vi "BRig_RT__Case_Exp__State_initTrial2__v3.vi"(0 "input_dataCurrent":u16[](array[numeric]), 1 "input_dataTrial":u16[][](array[numeric]), 3 "input_dataExp":u16[](array[numeric]), 6 "input_dataBlock":u16[][](array[numeric]), 8 "input_dataLC":u16[](array[numeric])) -> (7 "output_L_Wrong_Laser_l2":bool, 9 "output_L_Wrong_Event_l2":bool, 10 "output_L_Power_l1":dbl, 11 "output_L_Reward_Laser_l2":bool, 12 "output_L_Power_l2":dbl, 13 "output_L_Reward_Event_l2":bool, 14 "output_dataCurrent":u16[](array[numeric]), 15 "output_dataTrial":u16[][](array[numeric]), 16 "output_L_Reward_Event_l1":bool, 17 "output_L_Reward_Laser_l1":bool, 18 "output_L_Wrong_Event_l1":bool, 19 "output_L_Wrong_Laser_l1":bool)   [LabVIEW 2014]
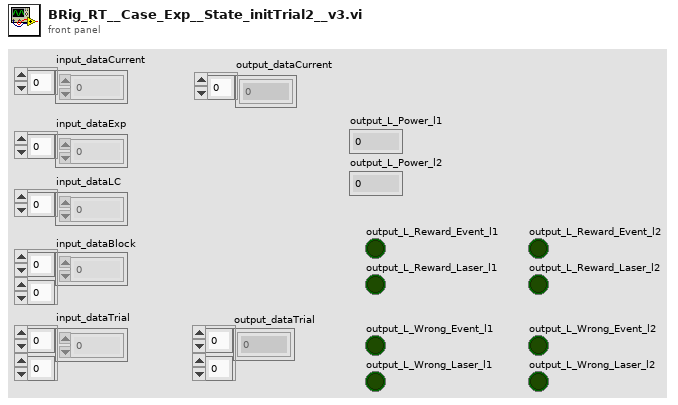
[diagram p1: front panel]
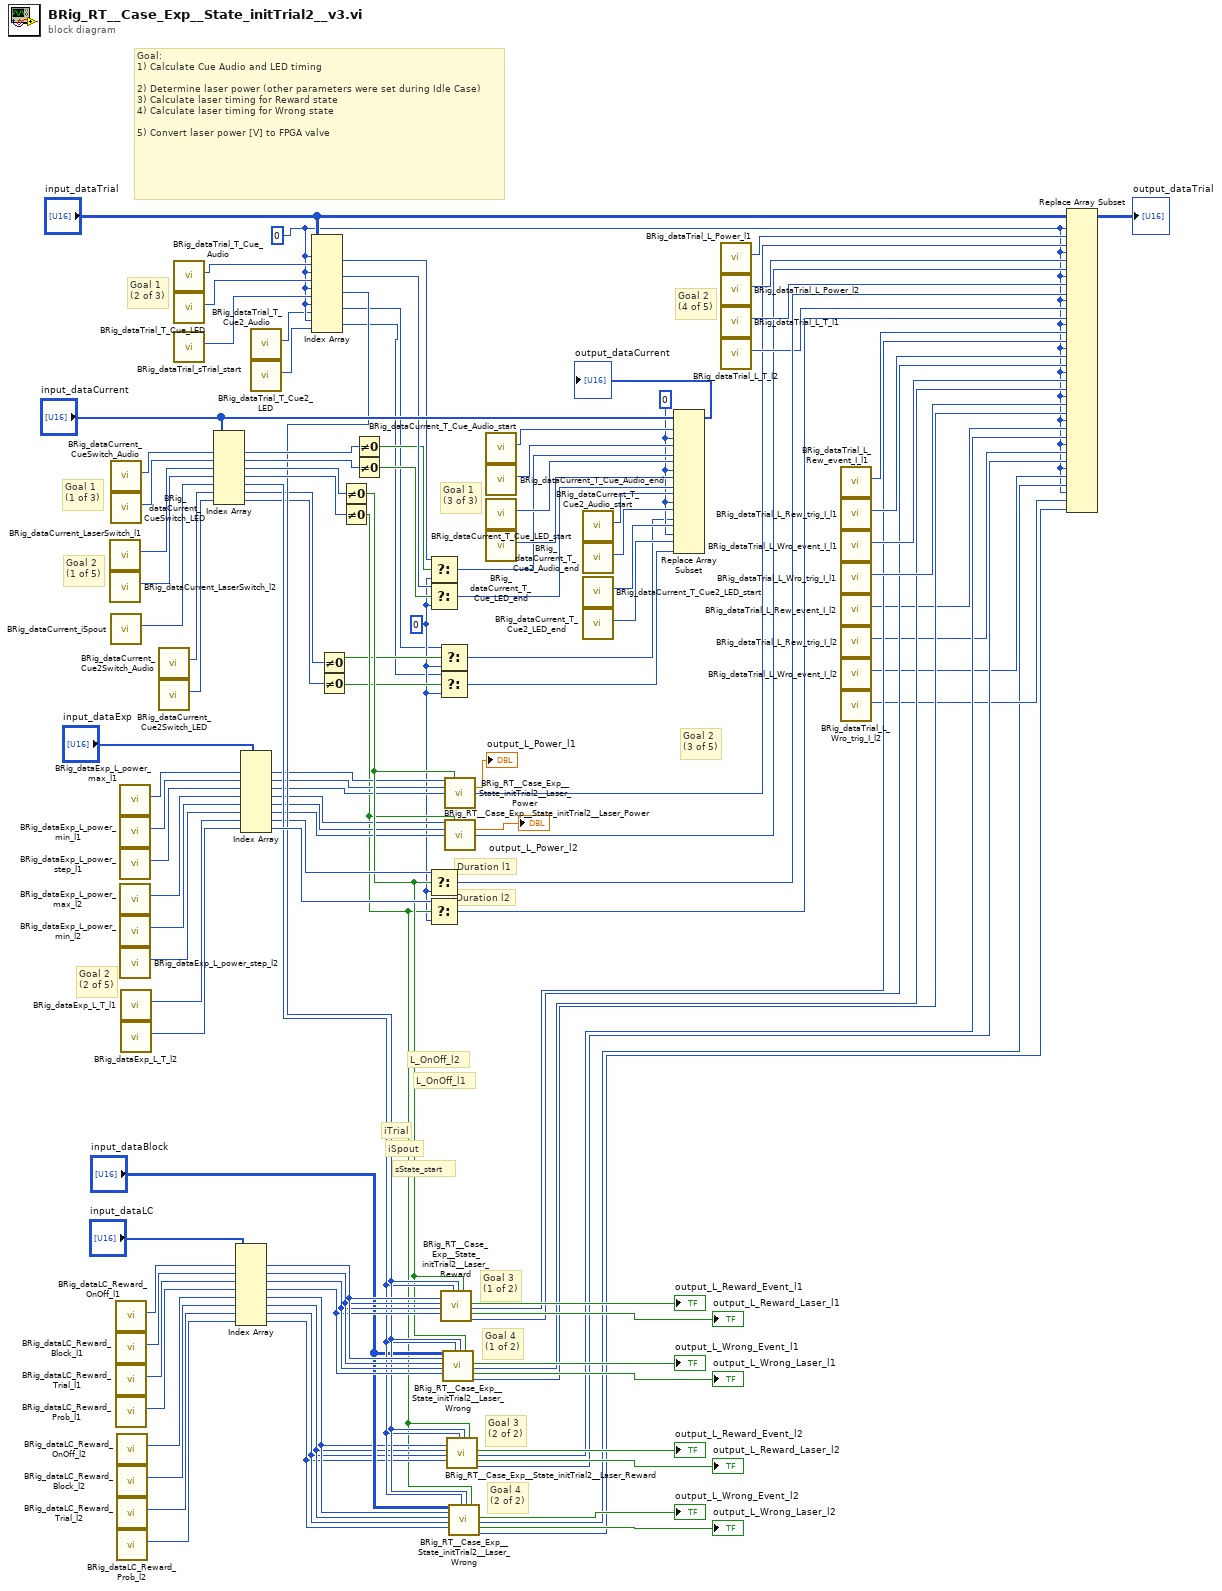
[diagram p0: block diagram]
diagram:
  w19 = 0
  w10 = u16 0 ("f")
  w3 = u16 0 ("new element/subarray")
  # "L_OnOff_l2"
  # "Goal 2\n(3 of 5)"
  # "Goal 4\n(2 of 2)"
  # "Goal 4\n(1 of 2)"
  # "Goal 3\n(2 of 2)"
  # "Goal 3\n(1 of 2)"
  # "L_OnOff_l1"
  # "iTrial"
  # "sState_start"
  # "iSpout"
  # "Goal 2\n(4 of 5)"
  # "Goal 2\n(2 of 5)"
  # "Duration l2"
  # "Duration l1"
  # "Goal 2\n(1 of 5)"
  # "Goal 1\n(3 of 3)"
  # "Goal 1\n(2 of 3)"
  # "Goal 1\n(1 of 3)"
  # "Goal:\n1) Calculate Cue Audio and LED timing\n\n2) Determine laser power (other parameters were set during Idle Case)\n3) Calculate laser timing for Reward state\n4) Calculate laser timing for Wrong state\n\n5) Convert laser power [V] to FPGA valve"
  n1 = call "BRig_dataCurrent_LaserSwitch_l1.vi"() -> ("output_LaserSwitch_l1"=w103:i32)  [unwired: 11 in]
  n2 = call "BRig_dataCurrent_LaserSwitch_l2.vi"() -> ("output_LaserSwitch_l2"=w102:i32)  [unwired: 11 in]
  n3 = call "BRig_dataCurrent_CueSwitch_Audio.vi"() -> ("output_CueSwitch_Audio"=w118:i32)  [unwired: 11 in]
  n4 = call "BRig_dataCurrent_CueSwitch_LED.vi"() -> ("output_CueSwitch_LED"=w116:i32)  [unwired: 11 in]
  n5 = call "BRig_dataCurrent_iSpout.vi"() -> ("output_iSpout"=w73:i32)  [unwired: 11 in]
  n6 = call "BRig_dataLC_Reward_OnOff_l1.vi"() -> ("output_Reward_OnOff"=w79:i32)  [unwired: 11 in]
  n7 = call "BRig_dataLC_Reward_Block_l1.vi"() -> ("output_Reward_Block"=w78:i32)  [unwired: 11 in]
  n8 = call "BRig_dataLC_Reward_Trial_l1.vi"() -> ("output_Reward_Trial"=w77:i32)  [unwired: 11 in]
  n9 = call "BRig_dataLC_Reward_Prob_l1.vi"() -> ("output_Reward_Prob"=w76:i32)  [unwired: 11 in]
  n10 = call "BRig_dataLC_Reward_OnOff_l2.vi"() -> ("output_Reward_OnOff_l2"=w67:i32)  [unwired: 11 in]
  n11 = call "BRig_dataLC_Reward_Block_l2.vi"() -> ("output_Reward_Block_l2"=w66:i32)  [unwired: 11 in]
  n12 = call "BRig_dataLC_Reward_Trial_l2.vi"() -> ("output_Reward_Trial_l2"=w65:i32)  [unwired: 11 in]
  n13 = call "BRig_dataLC_Reward_Prob_l2.vi"() -> ("output_Reward_Prob_l2"=w64:i32)  [unwired: 11 in]
  n14 = call "BRig_dataExp_L_power_max_l1.vi"() -> ("output_L_power_max_l1"=w100:i32)  [unwired: 11 in]
  n15 = call "BRig_dataExp_L_power_min_l1.vi"() -> ("output_L_power_min_l1"=w99:i32)  [unwired: 11 in]
  n16 = call "BRig_dataExp_L_power_step_l1.vi"() -> ("output_L_power_step_l1"=w98:i32)  [unwired: 11 in]
  n17 = call "BRig_dataExp_L_power_max_l2.vi"() -> ("output_L_power_max_l2"=w97:i32)  [unwired: 11 in]
  n18 = call "BRig_dataExp_L_power_min_l2.vi"() -> ("output_L_power_min_l2"=w96:i32)  [unwired: 11 in]
  n19 = call "BRig_dataExp_L_power_step_l2.vi"() -> ("output_L_power_step_l2"=w95:i32)  [unwired: 11 in]
  n20 = call "BRig_dataExp_L_T_l1.vi"() -> ("output_L_T_l1"=w94:i32)  [unwired: 11 in]
  n21 = call "BRig_dataExp_L_T_l2.vi"() -> ("output_L_T_l2"=w93:i32)  [unwired: 11 in]
  n22 = call "BRig_dataCurrent_Cue2Switch_Audio.vi"() -> ("output_Cue2Switch_Audio"=w16:i32)  [unwired: 11 in]
  n23 = call "BRig_dataCurrent_Cue2Switch_LED.vi"() -> ("output_Cue2Switch_LED"=w15:i32)  [unwired: 11 in]
  n24 = call "BRig_dataTrial_T_Cue_Audio.vi"() -> ("output_T_Cue_Audio"=w108:i32)  [unwired: 11 in]
  n25 = call "BRig_dataTrial_T_Cue_LED.vi"() -> ("output_T_Cue_LED"=w107:i32)  [unwired: 11 in]
  n26 = call "BRig_dataTrial_sTrial_start.vi"() -> ("output_sTrial_start"=w72:i32)  [unwired: 11 in]
  n27 = Index Array(array="input_dataCurrent", index #1=w118, index #2=w116, index #3=w103, index #4=w102, index #5=w73, index #6=w16, index #7=w15) -> (element #1=w111:u16, element #2=w110:u16, element #3=w75:u16, element #4=w74:u16, element #5=w62:u16, element #6=w14:u16, element #7=w13:u16)
  n28 = Index Array(array="input_dataLC", index #1=w79, index #2=w78, index #3=w77, index #4=w76, index #5=w67, index #6=w66, index #7=w65, index #8=w64) -> (element #1=w71:u16, element #2=w70:u16, element #3=w69:u16, element #4=w68:u16, element #5=w60:u16, element #6=w59:u16, element #7=w58:u16, element #8=w57:u16)
  n29 = Index Array(array="input_dataExp", index #1=w100, index #2=w99, index #3=w98, index #4=w97, index #5=w96, index #6=w95, index #7=w94, index #8=w93) -> (element #1=w30:u16, element #2=w29:u16, element #3=w28:u16, element #4=w25:u16, element #5=w24:u16, element #6=w23:u16, element #7=w32:u16, element #8=w90:u16)
  n30 = call "BRig_dataTrial_T_Cue2_Audio.vi"() -> ("output_T_Cue2_Audio"=w18:i32)  [unwired: 11 in]
  n31 = call "BRig_dataTrial_T_Cue2_LED.vi"() -> ("output_T_Cue2_LED"=w17:i32)  [unwired: 11 in]
  n32 = Index Array(array="input_dataTrial", index (row) #1=w19, index (col) #1=w108, index (row) #2=w19, index (col) #2=w107, index (row) #3=w19, index (col) #3=w72, index (row) #4=w19, index (col) #4=w18, index (row) #5=w19, index (col) #5=w17) -> (element #1=w106:u16, element #2=w105:u16, element #3=w63:u16, element #4=w9:u16, element #5=w8:u16)
  n33 = Not Equal To 0?(x=w14) -> (x != 0?=w12:bool)
  n34 = Not Equal To 0?(x=w13) -> (x != 0?=w11:bool)
  n35 = Not Equal To 0?(x=w75) -> (x != 0?=w31:bool)
  n36 = Not Equal To 0?(x=w74) -> (x != 0?=w22:bool)
  n37 = Not Equal To 0?(x=w111) -> (x != 0?=w92:bool)
  n38 = Not Equal To 0?(x=w110) -> (x != 0?=w91:bool)
  n39 = Select(t=w106, s=w92, f=w10) -> (s? t:f=w109:u16)
  n40 = Select(t=w105, s=w91, f=w10) -> (s? t:f=w104:u16)
  n41 = Select(t=w32, s=w31, f=w10) -> (s? t:f=w83:u16)
  n42 = Select(t=w90, s=w22, f=w10) -> (s? t:f=w81:u16)
  n43 = Select(t=w9, s=w12, f=w10) -> (s? t:f=w2:u16)
  n44 = Select(t=w8, s=w11, f=w10) -> (s? t:f=w1:u16)
  n45 = call "BRig_RT__Case_Exp__State_initTrial2__Laser_Reward.vi"("input_L_OnOff"=w71, "input_L_Block"=w70, "input_L_Trial"=w69, "input_L_Probability"=w68, "input_iSpout"=w62, "input_sState_start"=w63, "input_LaserSwitch"=w31) -> ("output_LR_Event"=→"output_L_Reward_Event_l1":bool, "output_LR_Event_num"=w44:u16, "output_LR_Laser"=→"output_L_Reward_Laser_l1":bool, "output_LR_Laser_num"=w43:u16)  [unwired: 9 in]
  n46 = call "BRig_RT__Case_Exp__State_initTrial2__Laser_Wrong.vi"("input_dataBlock"="input_dataBlock", "input_L_OnOff"=w71, "input_L_Block"=w70, "input_L_Trial"=w69, "input_L_Probability"=w68, "input_iSpout"=w62, "input_sState_start"=w63, "input_LaserSwitch"=w31) -> ("output_LR_Event"=→"output_L_Wrong_Event_l1":bool, "output_LR_Event_num"=w42:u16, "output_LR_Laser"=→"output_L_Wrong_Laser_l1":bool, "output_LR_Laser_num"=w41:u16)  [unwired: 8 in]
  n47 = call "BRig_RT__Case_Exp__State_initTrial2__Laser_Power.vi"("input_L_Power_max__x100"=w30, "input_LaserSwitch"=w31, "input_L_Power_min__x100"=w29, "input_L_Power_step__x100"=w28) -> ("output_L_Power"=→"output_L_Power_l1":dbl, "output_L_Power_x100"=w26:u16)  [unwired: 10 in]
  n48 = call "BRig_RT__Case_Exp__State_initTrial2__Laser_Power.vi"("input_L_Power_max__x100"=w25, "input_LaserSwitch"=w22, "input_L_Power_min__x100"=w24, "input_L_Power_step__x100"=w23) -> ("output_L_Power"=→"output_L_Power_l2":dbl, "output_L_Power_x100"=w20:u16)  [unwired: 10 in]
  n49 = call "BRig_RT__Case_Exp__State_initTrial2__Laser_Reward.vi"("input_L_OnOff"=w60, "input_L_Block"=w59, "input_L_Trial"=w58, "input_L_Probability"=w57, "input_iSpout"=w62, "input_sState_start"=w63, "input_LaserSwitch"=w22) -> ("output_LR_Event"=→"output_L_Reward_Event_l2":bool, "output_LR_Event_num"=w39:u16, "output_LR_Laser"=→"output_L_Reward_Laser_l2":bool, "output_LR_Laser_num"=w37:u16)  [unwired: 9 in]
  n50 = call "BRig_RT__Case_Exp__State_initTrial2__Laser_Wrong.vi"("input_dataBlock"="input_dataBlock", "input_L_OnOff"=w60, "input_L_Block"=w59, "input_L_Trial"=w58, "input_L_Probability"=w57, "input_iSpout"=w62, "input_sState_start"=w63, "input_LaserSwitch"=w22) -> ("output_LR_Event"=→"output_L_Wrong_Event_l2":bool, "output_LR_Event_num"=w34:u16, "output_LR_Laser"=→"output_L_Wrong_Laser_l2":bool, "output_LR_Laser_num"=w33:u16)  [unwired: 8 in]
  n51 = call "BRig_dataCurrent_T_Cue_Audio_start.vi"() -> ("output_T_Cue_Audio_start"=w115:i32)  [unwired: 11 in]
  n52 = call "BRig_dataCurrent_T_Cue_Audio_end.vi"() -> ("output_T_Cue_Audio_end"=w114:i32)  [unwired: 11 in]
  n53 = call "BRig_dataCurrent_T_Cue_LED_start.vi"() -> ("output_T_Cue_LED_start"=w113:i32)  [unwired: 11 in]
  n54 = call "BRig_dataCurrent_T_Cue_LED_end.vi"() -> ("output_T_Cue_LED_end"=w112:i32)  [unwired: 11 in]
  n55 = call "BRig_dataCurrent_T_Cue2_Audio_start.vi"() -> ("output_T_Cue2_Audio_start"=w7:i32)  [unwired: 11 in]
  n56 = call "BRig_dataCurrent_T_Cue2_Audio_end.vi"() -> ("output_T_Cue2_Audio_end"=w6:i32)  [unwired: 11 in]
  n57 = call "BRig_dataCurrent_T_Cue2_LED_start.vi"() -> ("output_T_Cue2_LED_start"=w5:i32)  [unwired: 11 in]
  n58 = call "BRig_dataCurrent_T_Cue2_LED_end.vi"() -> ("output_T_Cue2_LED_end"=w4:i32)  [unwired: 11 in]
  n59 = Replace Array Subset(array="input_dataCurrent", new element #1=w3, index #1=w115, new element #2=w109, index #2=w114, new element #3=w3, index #3=w113, new element #4=w104, index #4=w112, new element #5=w3, index #5=w7, new element #6=w2, index #6=w6, new element #7=w3, index #7=w5, new element #8=w1, index #8=w4) -> (→"output_dataCurrent":u16[])
  n60 = call "BRig_dataTrial_L_Power_l1.vi"() -> ("output_L_Power_l1"=w86:i32)  [unwired: 11 in]
  n61 = call "BRig_dataTrial_L_Power_l2.vi"() -> ("output_L_Power_l2"=w85:i32)  [unwired: 11 in]
  n62 = call "BRig_dataTrial_L_T_l1.vi"() -> ("output_L_T_l1"=w84:i32)  [unwired: 11 in]
  n63 = call "BRig_dataTrial_L_T_l2.vi"() -> ("output_L_T_l2"=w82:i32)  [unwired: 11 in]
  n64 = call "BRig_dataTrial_L_Rew_event_I_l1.vi"() -> ("output_L_Rew_event_I_l1"=w52:i32)  [unwired: 11 in]
  n65 = call "BRig_dataTrial_L_Rew_trig_I_l1.vi"() -> ("output_L_Rew_trig_I_l1"=w51:i32)  [unwired: 11 in]
  n66 = call "BRig_dataTrial_L_Wro_event_I_l1.vi"() -> ("output_L_Wro_event_I_l1"=w50:i32)  [unwired: 11 in]
  n67 = call "BRig_dataTrial_L_Wro_trig_I_l1.vi"() -> ("output_L_Wro_trig_I_l1"=w49:i32)  [unwired: 11 in]
  n68 = call "BRig_dataTrial_L_Rew_event_I_l2.vi"() -> ("output_L_Rew_event_I_l2"=w40:i32)  [unwired: 11 in]
  n69 = call "BRig_dataTrial_L_Rew_trig_I_l2.vi"() -> ("output_L_Rew_trig_I_l2"=w38:i32)  [unwired: 11 in]
  n70 = call "BRig_dataTrial_L_Wro_event_I_l2.vi"() -> ("output_L_Wro_event_I_l2"=w36:i32)  [unwired: 11 in]
  n71 = call "BRig_dataTrial_L_Wro_trig_I_l2.vi"() -> ("output_L_Wro_trig_I_l2"=w35:i32)  [unwired: 11 in]
  n72 = Replace Array Subset(array="input_dataTrial", new element #1=w26, index (row) #1=w19, index (col) #1=w86, new element #2=w20, index (row) #2=w19, index (col) #2=w85, new element #3=w83, index (row) #3=w19, index (col) #3=w84, new element #4=w81, index (row) #4=w19, index (col) #4=w82, new element #5=w44, index (row) #5=w19, index (col) #5=w52, new element #6=w43, index (row) #6=w19, index (col) #6=w51, new element #7=w42, index (row) #7=w19, index (col) #7=w50, new element #8=w41, index (row) #8=w19, index (col) #8=w49, new element #9=w39, index (row) #9=w19, index (col) #9=w40, new element #10=w37, index (row) #10=w19, index (col) #10=w38, new element #11=w34, index (row) #11=w19, index (col) #11=w36, new element #12=w33, index (row) #12=w19, index (col) #12=w35) -> (→"output_dataTrial":u16[][])
